vi "fastscan graph.vi"(6 "x pts flyback":i32, 7 "Samples to Average":i32, 9 "x max":dbl, 10 "x min":dbl, 11 "x pixels":i32) -> (3 "Array":dbl[](array[numeric]))   [LabVIEW 2012]
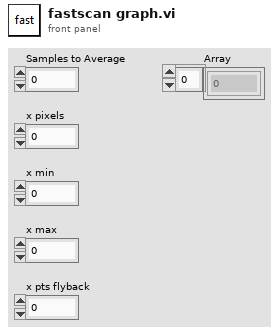
[diagram p1: front panel]
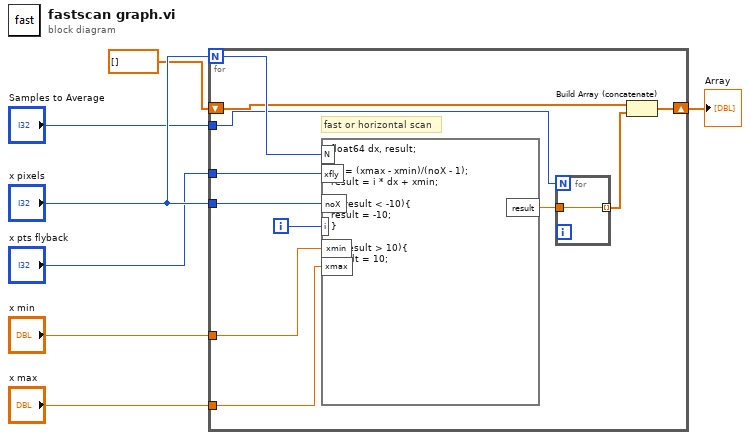
[diagram p0: block diagram]
diagram:
  n1 = for {
    N: "x pixels" -> [w13]
    tunnel: "x min" -> [w17]
    tunnel: "x max" -> [w16]
    tunnel: "x pixels" -> [w15]
    tunnel: "x pts flyback" -> [w14]
    tunnel: "Samples to Average" -> [w11]
    shift-right: [w8] -> w7
    shift-left: dbl[] [] -> [w9]
    i -> [w18]
    # "fast or horizontal scan"
    n2 = formula code="float64 dx, result;\n\ndx = (xmax - xmin)/(noX - 1);\nresult = i * dx + xmin;\n\nif (result < -10){\nresult = -10;\n}\n\nif (result > 10){\nresult = 10;\n}"("i"=w18, "xmin"=w17, "xmax"=w16, "noX"=w15, "xfly"=w14, "N"=w13) -> ("result"=w12:dbl)
    n3 = for {
      N: w11 -> [_]
      tunnel: w12 -> [w19]
      tunnel: [w19] -> w10 mode=indexing
    }
    n4 = Build Array (concatenate)(w9, w10) -> (w8:dbl[])
  }
  "Array" <- w7
